vi "Update Package Version.vi"(8 "error in (no error)":errorcluster, 11 "Build Package Step in":refnum<class "Build VIPB Step.lvclass">) -> (0 "error out":errorcluster, 3 "Build Package Step out":refnum<class "Build VIPB Step.lvclass">)   [LabVIEW 2019, in "VIPM.lvlib" / "Build VIPB Step.lvclass"]
uses:
  Build VIPB Step.lvclass
  C:/Users/pasca/source/repos/mgi-solution-explorer-extensions/libs/Solution.lvlibp/Solution/Build Item/Build Step.lvclass
  Build VIPB Step.lvclass/Build VIPB Step.ctl
  libs/Solution.lvlibp/Solution/Build Item/Read Settings.vi
  <vilib>/JKI/VIPM API/VIPM API_vipm_api.lvlib
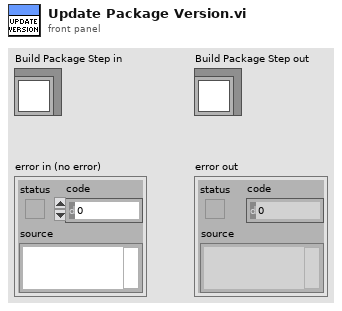
[diagram p1: front panel]
types:
  T1 = typedef "Solution.lvlibp/Build Step.lvclass/Build Settings.ctl" = cluster{"Force?":bool, "Version":T2}
  T2 = typedef "Solution.lvlibp/Version.ctl" = cluster{"Major":i32, "Minor":i32, "Build":i32, "Patch":i32}
  T3 = typedef "VIPM API_vipm_api.lvlib/VI Package Build Spec Data Cluster_vipm_api.ctl" = cluster{"Package Version":T4, "Product Name":string, "Company Name":string, "Author Name (Person or Company)":string, "Product Homepage (URL)":string, "Legal Copyright":string, "License Agreement Name":string, "Product Description Summary":string, "Product Description":string, "Release Notes - Change Log":string}
  T4 = typedef "VIPM API_vipm_api.lvlib/Version Info Cluster_vipm_api.ctl" = cluster{"major":u32, "minor":u32, "patch":u32, "build":u32}
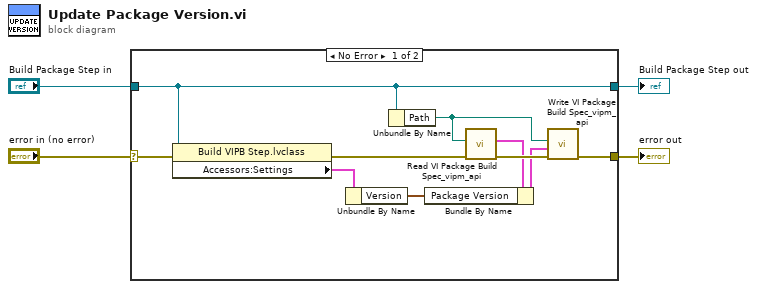
[diagram p0: block diagram]
diagram:
  n1 = case shown="No Error" "error in (no error)" {
    selector: "error in (no error)" -> [w14 w16]
    tunnel: [w12 w16] -> w3
    tunnel: [w10 w15] -> w1
    tunnel: "Build Package Step in" -> [w10 w15]
    frame No Error {
      n2 = property class="Build VIPB Step.lvclass"(reference=w10, error in=w14) -> (error out=w11:errorcluster, "Accessors:Settings"=w6:T1)  [unwired: 1 out]
      n3 = Unbundle By Name(w6) -> ("Version"=w5:T2)
      n4 = Unbundle By Name(w10) -> ("Path"=w7:path)
      n5 = call <vilib>:"Read VI Package Build Spec_vipm_api.vi"("error in (no error)"=w11, "Path to VIPB File"=w7) -> ("error out"=w13:errorcluster, "VI Package Build Spec Data"=w9:T3)  [unwired: 8 in]
      n6 = Bundle By Name(cluster=w9, "Package Version"=w5) -> (w8:T3)
      n7 = call <vilib>:"Write VI Package Build Spec_vipm_api.vi"("error in (no error)"=w13, "VI Package Build Spec Data"=w8, "Path to VIPB File"=w7) -> ("error out"=w12:errorcluster)  [unwired: 8 in]
    }
    frame Error {
    }
  }
  "error out" <- w3
  "Build Package Step out" <- w1
